vi "Stop Iterations.vi"(8 "error in (no error)":errorcluster, 11 "Iterator Actor in":refnum<class "Iterator Actor.lvclass">) -> (0 "error out":errorcluster, 3 "Iterator Actor out":refnum<class "Iterator Actor.lvclass">)   [LabVIEW 2017, in "Iterator Actor.lvlib" / "Iterator Actor.lvclass"]
doc: "Stops all the subsequent iterations."
uses:
  Iterator Actor.lvclass
  Iterator Actor.lvclass/Iterator Actor.ctl
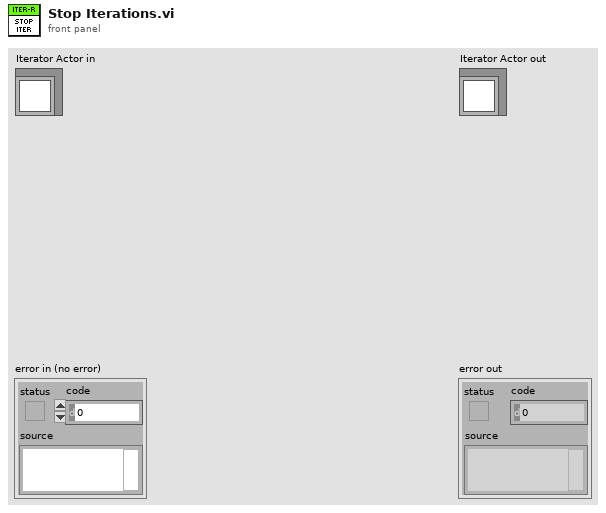
[diagram p1: front panel]
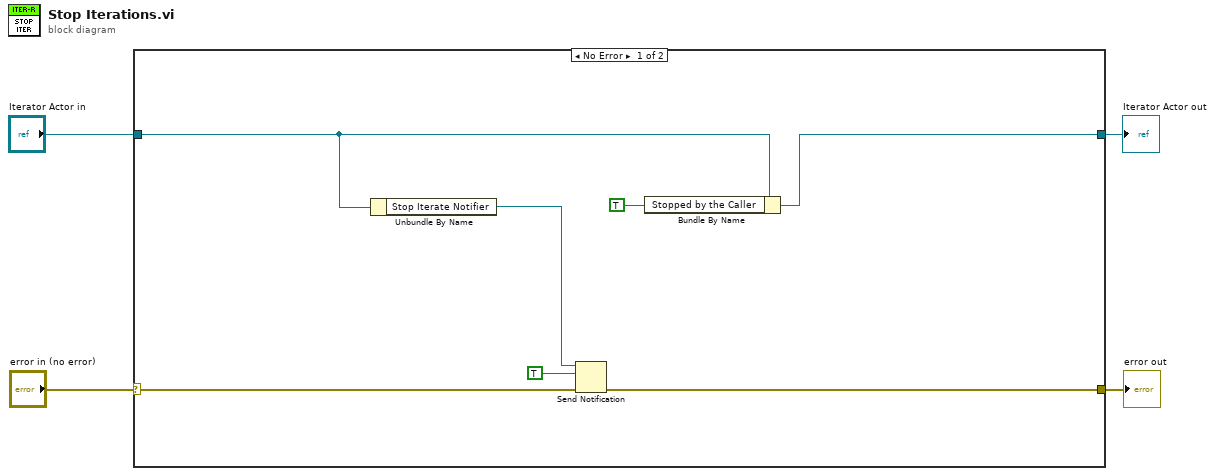
[diagram p0: block diagram]
diagram:
  n1 = case shown="No Error" "error in (no error)" {
    selector: "error in (no error)" -> [w10 w13]
    tunnel: [w11 w13] -> w3
    tunnel: [w6 w12] -> w1
    tunnel: "Iterator Actor in" -> [w7 w12]
    frame No Error {
      n2 = Unbundle By Name(w7) -> ("Stop Iterate Notifier"=w9:refnum<notifier>)
      n3 = Send Notification(notification=TRUE, notifier=w9, error in (no error)=w10) -> (error out=w11:errorcluster)  [unwired: 1 out]
      n4 = Bundle By Name(cluster=w7, "Stopped by the Caller"=TRUE) -> (w6:refnum<class "Iterator Actor.lvclass">)
    }
    frame Error {
    }
  }
  "error out" <- w3
  "Iterator Actor out" <- w1
